vi "get_moving_by_name.vi"(8 "error in (no error)":errorcluster caption="错误输入（无错误）", 10 "name":string, 11 "MotorSystem输入":refnum<class "MotorSystem.lvclass">) -> (0 "error out":errorcluster caption="错误输出", 2 "moving?":bool, 3 "MotorSystem输出":refnum<class "MotorSystem.lvclass">)   [LabVIEW 2016, in "MotionControl_UFO_3DOF.lvlib" / "MotorSystem.lvclass"]
uses:
  <userlib>/MotionControl_UFO_3DOF/MotorSystem/MotorSystem.lvclass
  <userlib>/MotionControl_UFO_3DOF/MotorSystem/MotorSystem.lvclass/MotorSystem.ctl
  <userlib>/MotionControl_UFO_3DOF/OneMotion/OneMotion.lvclass
  <userlib>/MotionControl_UFO_3DOF/StepMotor/StepMotor.lvclass
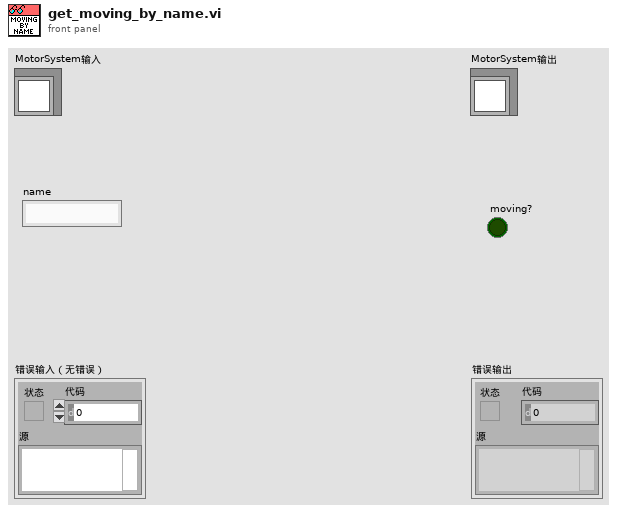
[diagram p1: front panel]
types:
  T1 = typedef "MotionControl_UFO_3DOF.lvlib/MotorSystem.lvclass/MotionCluster.ctl" = cluster{"OneMotion.lvclass":refnum<class "OneMotion.lvclass">, "connected?":bool, "default enabled?":bool, "enabled?":bool}
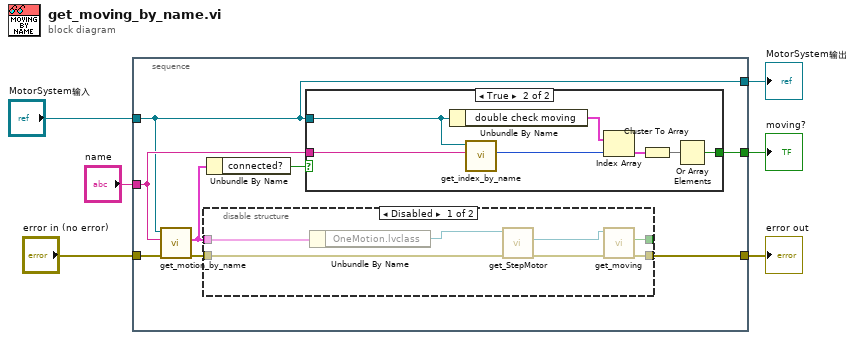
[diagram p0: block diagram]
diagram:
  n1 = stacked-sequence {
    tunnel: [w12] -> w6
    tunnel: "MotorSystem输入" -> [w8]
    tunnel: "name" -> [w9]
    tunnel: "error in (no error)" -> [w14]
    tunnel: [w7] -> w2
    tunnel: [w8] -> w1
    frame #0 {
      n2 = call <userlib>:"get_motion_by_name.vi"("error in (no error)"=w14, "name"=w9, "MotorSystem in"=w8) -> ("error out"=w13:errorcluster, "motion cluster"=w11:T1)  [unwired: 6 in, 1 out]
      n3 = disable-structure shown="Disabled" {
        disable-tunnel: w11 -> [w28 _]
        disable-tunnel: w13 -> [w25 _]
        disable-tunnel: [w23 _] -> w12
        disable-tunnel: [w22 _] -> _
        frame Disabled {
          n4 = Unbundle By Name(w28) -> ("OneMotion.lvclass"=w27:refnum<class "OneMotion.lvclass">)
          n5 = call <userlib>:"get_StepMotor.vi"("error in (no error)"=w25, "OneMotion输入"=w27) -> ("error out"=w24:errorcluster, "StepMotor.lvclass"=w26:refnum<class "StepMotor.lvclass">)  [unwired: 7 in, 1 out]
          n6 = call <userlib>:"get_moving.vi"("error in (no error)"=w24, "StepMotor输入"=w26) -> ("error out"=w23:errorcluster, "moving?"=w22:bool)  [unwired: 7 in, 1 out]
        }
        frame Enabled {
        }
      }
      n7 = Unbundle By Name(w11) -> ("connected?"=w10:bool)
      n8 = case shown="True" w10 {
        tunnel: w9 -> [_ w19]
        tunnel: w8 -> [_ w18]
        tunnel: [_ w15] -> w7
        frame False {
        }
        frame True {
          n9 = Unbundle By Name(w18) -> ("double check moving"=w20:cluster{"1st check":bool, "2nd check":bool}[])
          n10 = call <userlib>:"get_index_by_name.vi"("name"=w19, "MotorSystem 输入"=w18) -> ("index (0-based)"=w21:u32)  [unwired: 7 in, 2 out]
          n11 = Index Array(array=w20, index=w21) -> (element=w17:cluster{"1st check":bool, "2nd check":bool})
          n12 = Cluster To Array(cluster=w17) -> (array=w16:bool[])
          n13 = Or Array Elements(Boolean array=w16) -> (logical OR=w15:bool)
        }
      }
    }
  }
  "error out" <- w6
  "MotorSystem输出" <- w1
  "moving?" <- w2
